vi "Get LV Language.vi"() -> (1 "Language":T1=9 caption="Lang" items=["English"=9, "German"=7, "French"=12, "Japanese"=17, "Korean"=18, "Chinese (Simplified)"=2052])   [LabVIEW 2020]
uses:
  <vilib>/AppBuilder/CodeSignAPI/sTypeDef_Languages.ctl
  <resource>/Framework/Providers/Builds/Installer/CDK_sTypeDef_Languages.ctl
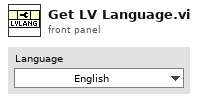
[diagram p1: front panel]
types:
  T1 = typedef "sTypeDef_Languages.ctl" = u16
  T2 = typedef "CDK_sTypeDef_Languages.ctl" = u16
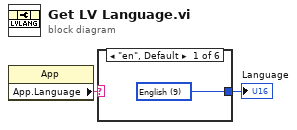
[diagram p0: block diagram]
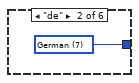
[diagram p2: hidden frame]
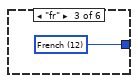
[diagram p3: hidden frame]
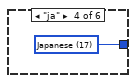
[diagram p4: hidden frame]
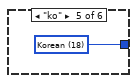
[diagram p5: hidden frame]
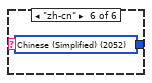
[diagram p6: hidden frame]
diagram:
  n1 = property class="App"() -> ("App.Language"=w1:string)  [unwired: 2 in, 2 out]
  n2 = case shown="\"en\", Default" w1 {
    tunnel: [w3 w4 w5 w6 w7 w8] -> w2
    frame "en", Default {
      w3 = T2 9 items=["English"=9, "German"=7, "French"=12, "Japanese"=17, "Korean"=18] ("Lang")
    }
    frame "de" {
      w4 = T2 7 items=["English"=9, "German"=7, "French"=12, "Japanese"=17, "Korean"=18] ("Lang")
    }
    frame "fr" {
      w5 = T2 12 items=["English"=9, "German"=7, "French"=12, "Japanese"=17, "Korean"=18] ("Lang")
    }
    frame "ja" {
      w6 = T2 17 items=["English"=9, "German"=7, "French"=12, "Japanese"=17, "Korean"=18] ("Lang")
    }
    frame "ko" {
      w7 = T2 18 items=["English"=9, "German"=7, "French"=12, "Japanese"=17, "Korean"=18] ("Lang")
    }
    frame "zh-cn" {
      w8 = T2 2052 items=["English"=9, "German"=7, "French"=12, "Japanese"=17, "Korean"=18, "Chinese (Simplified)"=2052] ("Lang")
    }
  }
  "Language" <- w2
